vi "Get DAQ tasks.vi"(8 "error in":errorcluster, 10 "Device Name":tag="Dev6", 11 "frequency":dbl=100.0 caption="Frecuencia PWM" format="%_6g") -> (0 "error out":errorcluster, 3 "Task list":T1)   [LabVIEW 2018]
uses:
  <vilib>/DAQmx/create/channels.llb/DAQmx Create Channel (DO-Digital Output).vi
  <vilib>/DAQmx/create/channels.llb/DAQmx Create Channel (CO-Pulse Generation-Frequency).vi
  <vilib>/DAQmx/configure/timing.llb/DAQmx Timing (Implicit).vi
  <vilib>/DAQmx/create/channels.llb/DAQmx Create Channel (AI-Voltage-Basic).vi
  typedef/Task list.ctl
  <vilib>/DAQmx/write.llb/DAQmx Write (Digital 1D Bool 1Chan 1Samp).vi
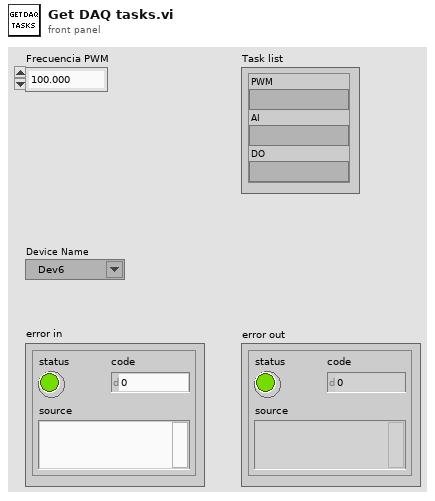
[diagram p1: front panel]
types:
  T1 = typedef "Task list.ctl" = cluster{"PWM":refnum<k21>, "AI":refnum<k21>, "DO":refnum<k21>}
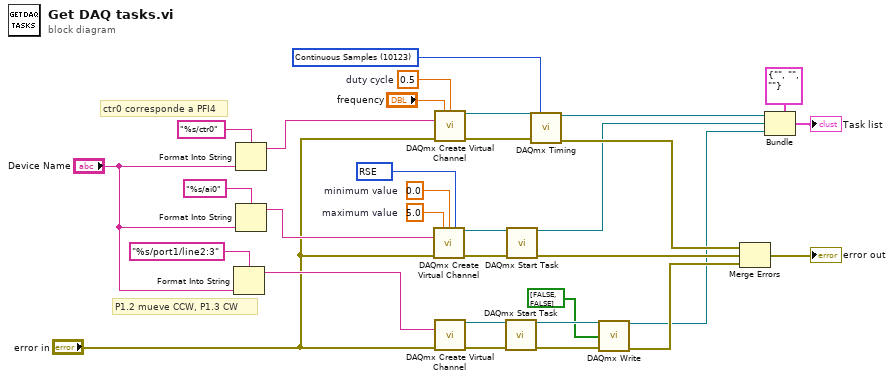
[diagram p0: block diagram]
diagram:
  w21 = 10083 items=["Default"=-1, "RSE"=10083, "NRSE"=10078, "Differential"=10106, "Pseudodifferential"=12529] ("input terminal configuration")
  w20 = 0.0  # minimum value
  w19 = 5.0  # maximum value
  w16 = 0.5  # duty cycle
  w12 = 10123 items=["Finite Samples"=10178, "Continuous Samples"=10123, "Hardware Timed Single Point"=12522] ("sample mode")
  # "P1.2 mueve CCW, P1.3 CW"
  # "ctr0 corresponde a PFI4"
  n1 = Format Into String(format string="%s/port1/line2:3", "Device Name") -> (resulting string=w32:string)  [unwired: 2 in, 1 out]
  n2 = Format Into String(format string="%s/ctr0", "Device Name") -> (resulting string=w29:string)  [unwired: 2 in, 1 out]
  n3 = Format Into String(format string="%s/ai0", "Device Name") -> (resulting string=w30:string)  [unwired: 2 in, 1 out]
  n4 = call-poly <vilib>:"DAQmx Create Virtual Channel.vi"("maximum value"=w19, "minimum value"=w20, "input terminal configuration"=w21, "physical channels"=w30, "error in"="error in") -> ("task out"=w24:refnum<k21>, "error out"=w23:errorcluster)  [unwired: 9 in]
  n5 = call-poly <vilib>:"DAQmx Create Virtual Channel.vi"("frequency"="frequency", "duty cycle"=w16, "counter"=w29, "error in"="error in") -> ("task out"=w14:refnum<k21>, "error out"=w13:errorcluster)  [unwired: 10 in]
  n6 = call-poly <vilib>:"DAQmx Create Virtual Channel.vi"("lines"=w32, "error in"="error in") -> ("task out"=w18:refnum<k21>, "error out"=w17:errorcluster)  [unwired: 12 in]
  n7 = call <vilib>:"DAQmx Start Task.vi"("task/channels in"=w18, "error in"=w17) -> ("task out"=w3:refnum<k21>, "error out"=w22:errorcluster)  [unwired: 12 in]
  n8 = call <vilib>:"DAQmx Start Task.vi"("task/channels in"=w24, "error in"=w23) -> ("task out"=w9:refnum<k21>, "error out"=w25:errorcluster)  [unwired: 12 in]
  n9 = call-poly <vilib>:"DAQmx Timing.vi"("task/channels in"=w14, "sample mode"=w12, "error in"=w13) -> ("task out"=w10:refnum<k21>, "error out"=w26:errorcluster)  [unwired: 11 in]
  n10 = call-poly <vilib>:"DAQmx Write.vi"("task/channels in"=w3, "data"=bool[] [FALSE, FALSE], "error in"=w22) -> ("task out"=w2:refnum<k21>, "error out"=w4:errorcluster)  [unwired: 10 in, 1 out]
  n11 = Merge Errors(w26, w25, w4) -> (→"error out":errorcluster)
  n12 = Bundle(cluster=T1 {"PWM"="", "AI"="", "DO"=""} ("Task list"), "PWM"=w10, "AI"=w9, "DO"=w2) -> (→"Task list":T1)
